vi "Air Density.vi"(11 "Temperature (K)":dbl) -> (3 "Density (kg/m^3)":dbl)   [LabVIEW 2019]
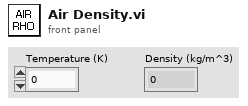
[diagram p1: front panel]
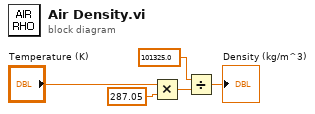
[diagram p0: block diagram]
diagram:
  n1 = Multiply(x="Temperature (K)", y=287.05) -> (x*y=w2:dbl)
  n2 = Divide(x=101325.0, y=w2) -> (x/y=→"Density (kg/m^3)":dbl)
